vi "set autorange.vi"(8 "error in (no error)":errorcluster, 10 "Auto Range (F: Off)":bool, 11 "VISA session":refnum<visa-resource-name>) -> (0 "error out":errorcluster, 3 "dup VISA session":refnum<visa-resource-name>)   [LabVIEW 2017]
panel:
  # "When autorange is set on, it also sets range to the middle value"
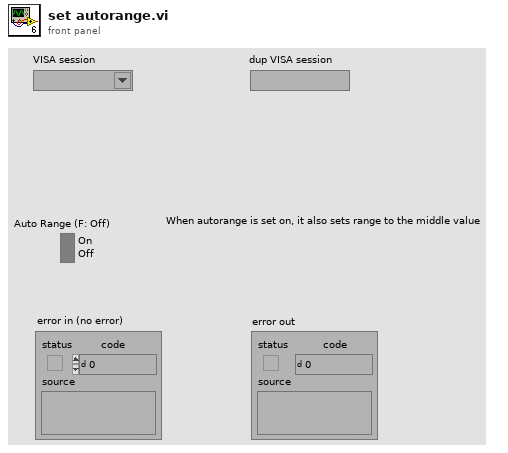
[diagram p1: front panel]
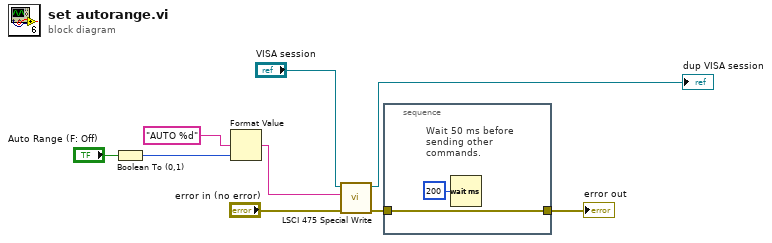
[diagram p0: block diagram]
diagram:
  n1 = Boolean To (0,1)(Boolean="Auto Range (F: Off)") -> (0, 1=w2:i16)
  n2 = Format Value(format string="AUTO %d", value (0)=w2) -> (output string=w1:string)  [unwired: 1 in]
  n3 = call "LSCI 475 Special Write.vi"("error in (no error)"="error in (no error)", "Write Buffer (\"\")"=w1, "VISA session"="VISA session") -> ("error out"=w6:errorcluster, "dup VISA session"=→"dup VISA session":refnum<visa-resource-name>)  [unwired: 6 in, 1 out]
  n4 = stacked-sequence {
    tunnel: w6 -> [w10]
    tunnel: [w10] -> w7
    frame #0 {
      # "Wait 50 ms before\nsending other\ncommands."
      n5 = Wait (ms)(milliseconds to wait=u32 200) -> ()  [unwired: 1 out]
    }
  }
  "error out" <- w7
